vi "Trial_Frame.vi"() -> ()   [LabVIEW 2012]
uses:
  <vilib>/nican/nican.llb/ncNetAttr.ctl
  <vilib>/nican/nican.llb/ncObjAttr.ctl
panel:
  in  "Data":u8[](array[numeric]) format="%.0x"
  in  "Data Length":u32
  in  "stop":bool
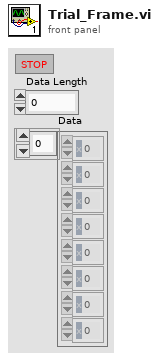
[diagram p1: front panel]
types:
  T1 = typedef "ncObjAttr.ctl" = cluster{"Period":u32, "Read Queue Length":u32, "Write Queue Length":u32, "Receive Changes Only":enum32{"FALSE", "TRUE"}, "Communication Type":enum32{"Receive Unsolicited", "Transmit Data By Call", "Receive Periodic Using Remote", "Transmit Data Periodically", "Receive By Call Using Remote", "Transmit By Response Only", "Transmit Periodic Waveform"}, "Transmit By Response":enum32{"FALSE", "TRUE"}, "Data Length":u32}
  T2 = typedef "ncNetAttr.ctl" = cluster{"Start On Open":enum32{"FALSE", "TRUE"}, "Baud Rate":u32, "Read Queue Length":u32, "Write Queue Length":u32, "Standard Comparator":u32, "Standard Mask":u32, "Extended Comparator":u32, "Extended Mask":u32}
  T3 = typedef "xobjhandle.ctl" = u32
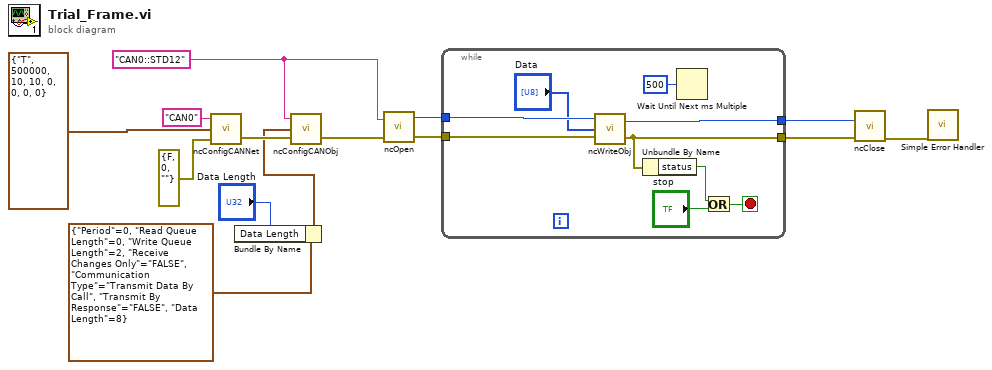
[diagram p0: block diagram]
diagram:
  w8 = "CAN0::STD12" ("ObjName")
  n1 = call <vilib>:"ncConfigCANNet.vi"("Error in"=errorcluster {"status"=FALSE, "code"=0, "source"=""}, "CAN Network Interface Config"=T2 {"Start On Open"=enum."TRUE", "Baud Rate"=500000, "Read Queue Length"=10, "Write Queue Length"=10, "Standard Comparator"=0, "Standard Mask"=0, "Extended Comparator"=0, "Extended Mask"=0}, "ObjName"="CAN0") -> ("Error out"=w13:errorcluster)  [unwired: 2 in]
  n2 = Bundle By Name(cluster=T1 {"Period"=0, "Read Queue Length"=0, "Write Queue Length"=2, "Receive Changes Only"=enum."FALSE", "Communication Type"=enum."Transmit Data By Call", "Transmit By Response"=enum."FALSE", "Data Length"=8} ("CAN Object Config"), "Data Length"="Data Length") -> (w4:T1)
  n3 = call <vilib>:"ncConfigCANObj.vi"("Error in"=w13, "CAN Object Config"=w4, "ObjName"=w8) -> ("Error out"=w12:errorcluster)  [unwired: 2 in]
  n4 = call <vilib>:"ncOpen.vi"("Error in"=w12, "ObjName"=w8) -> ("Error out"=w11:errorcluster, "ObjHandle out"=w2:T3)
  n5 = while {
    tunnel: w11 -> [w23]
    tunnel: [w16] -> w10
    tunnel: w2 -> [w19]
    tunnel: [w18] -> w1
    stop <- w21 stop-if-true
    n6 = call <vilib>:"ncWriteObj.vi"("Error in"=w23, "Data"="Data", "ObjHandle in"=w19) -> ("Error out"=w16:errorcluster, "ObjHandle out"=w18:T3)
    n7 = Unbundle By Name(w16) -> ("status"=w17:bool)
    n8 = Wait Until Next ms Multiple(millisecond multiple=u32 500) -> ()  [unwired: 1 out]
    n9 = Or(x=w17, y="stop") -> (x .or. y?=w21:bool)
  }
  n10 = call <vilib>:"ncClose.vi"("Error in"=w10, "ObjHandle in"=w1) -> ("Error out"=w9:errorcluster)  [unwired: 1 in]
  n11 = call <vilib>:"Simple Error Handler.vi"("error in (no error)"=w9) -> ()  [unwired: 4 in, 5 out]
